vi "Get BufferMap Status.vi"(8 "error in":errorcluster, 11 "BufferMap in":refnum<data-value>) -> (0 "error out":errorcluster, 1 "bufSize":i32, 2 "nbElements":i32, 3 "BufferMap":refnum<data-value>, 4 "full":bool, 5 "Names":string[](array[string]))   [LabVIEW 2013, in "CircularBuffer.lvlib" / "VariantBufferMap.lvclass"]
doc: "This VI returns data from the ring buffer starting from the oldest data and ending with the newest.\n\nThe data is duplicated at the output so this VI allocates new place in the memory for the output."
uses:
  VariantBufferMap.lvclass
  VariantBufferMap.lvclass/VariantBufferMap.ctl
  VariantBuffer/WriteBufferError.vi
  VariantBuffer/VariantBuffer.lvclass
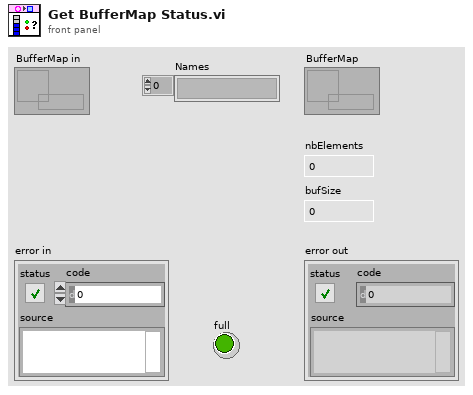
[diagram p1: front panel]
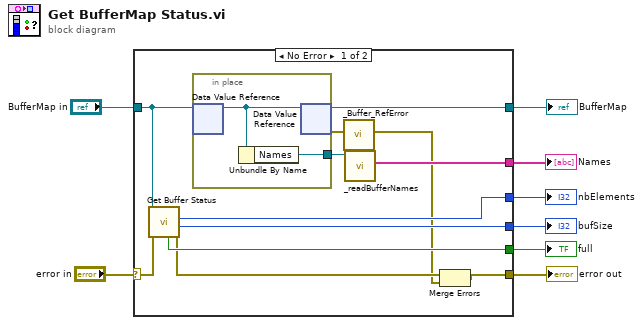
[diagram p0: block diagram]
diagram:
  n1 = case shown="No Error" "error in" {
    selector: "error in" -> [w12 w23]
    tunnel: "BufferMap in" -> [w18 w24]
    tunnel: [w20 w24] -> w7
    tunnel: [w19 w23] -> w4
    tunnel: [w17 _] -> w6
    tunnel: [w15 _] -> w3
    tunnel: [w16 _] -> w2
    tunnel: [w13 _] -> w1
    frame No Error {
      n2 = call "Get Buffer Status.vi"("error in"=w12, "Buffer in"=w18) -> ("error out"=w11:errorcluster, "bufSize"=w16:i32, "nbElements"=w17:i32, "full"=w15:bool)  [unwired: 5 in, 1 out]
      n3 = in-place {
        in-place-border: [w21] -> w14
        n4 = in-place-dvr #1(w18) -> (w22:refnum<class "VariantBufferMap.lvclass">)  [unwired: 1 out]
        n5 = Unbundle By Name(w22) -> ("Names"=w21:refnum<data-value>)
        n6 = in-place-dvr #1(w22) -> (w20:refnum<data-value>, w10:errorcluster)
      }
      n7 = call "_Buffer_RefError.vi"("error in (no error)"=w10) -> ("error out"=w9:errorcluster)  [unwired: 10 in]
      n8 = call "_readBufferNames.vi"("Data Value Reference in"=w14) -> ("Names"=w13:string[])  [unwired: 9 in, 1 out]
      n9 = Merge Errors(w11, w9) -> (w19:errorcluster)
    }
    frame Error {
    }
  }
  "error out" <- w4
  "BufferMap" <- w7
  "nbElements" <- w6
  "bufSize" <- w2
  "full" <- w3
  "Names" <- w1
